vi "Handle Error.vi"(8 "error in (no error)":errorcluster, 11 "cRIO-CO2 in":refnum<class "cRIO-CO2.lvclass">) -> (0 "error out":errorcluster, 2 "stop actor?":bool=TRUE, 3 "cRIO-CO2 out":refnum<class "cRIO-CO2.lvclass">)   [LabVIEW 2015, in "cRIO-Carbondioxide.lvlib" / "cRIO-CO2.lvlib" / "cRIO-CO2.lvclass"]
doc: "(<B>Filename</B>: Actor Framework.lvlib:Actor.lvclass:Handle Error.vi)\n\nDefines how the actor handles an error that occurred while processing a message.\n\nBy default, this method does nothing except stop the actor. This method also treats error code 43 (coming from <B>error in</B>) as a sign that the actor shut down normally. In this situation, the Handle Error method does not return the error on <B>error out</B>, meaning the actor's caller will not receive it. All other error codes will be returned on <B>error out</B>.\n\nA descendant class may override this method to change this behavior."
uses:
  cRIO-CO2.lvclass
  cRIO-CO2.lvclass/cRIO-CO2.ctl
  cRIO-CO2 Messages/Log Error Msg/Log Error Msg.lvclass/Log Error Msg.ctl
  <vilib>/ActorFramework/Message Enqueuer/Message Enqueuer.lvclass/Message Enqueuer.ctl
  <vilib>/ActorFramework/Message Enqueuer/Enqueue.vi
  <vilib>/ActorFramework/Message Priority Queue/Priority Enqueue.vi
  cRIO-CO2 Messages/Log Error Msg/Log Error Msg.lvclass
  <vilib>/ActorFramework/Actor/Actor.lvclass
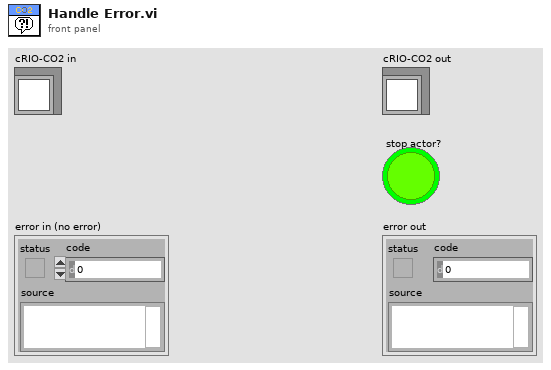
[diagram p1: front panel]
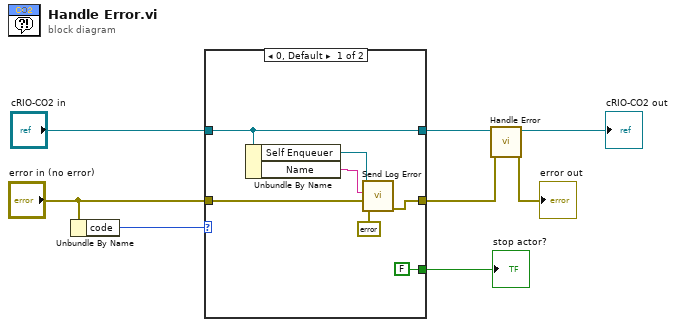
[diagram p0: block diagram]
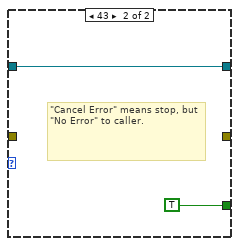
[diagram p2: hidden frame]
diagram:
  n1 = Unbundle By Name("error in (no error)") -> ("code"=w1:i32)
  n2 = case shown="0, Default" w1 {
    tunnel: "cRIO-CO2 in" -> [w11 w17]
    tunnel: [w11 w17] -> w5
    tunnel: [w9 _] -> w4
    tunnel: "error in (no error)" -> [w10 _]
    tunnel: [FALSE ("stop actor?") TRUE ("stop actor?")] -> w2
    frame 0, Default {
      n3 = Unbundle By Name(w11) -> ("Self Enqueuer"=w13:refnum<class "Message Enqueuer.lvclass">, "Name"=w12:string)
      n4 = call "Send Log Error.vi"("error in (no error)"=errorcluster {"status"=FALSE, "code"=0, "source"=""}, "error to log (no error)"=w10, "Source Name"=w12, "Message Enqueuer"=w13) -> ("error out"=w9:errorcluster)  [unwired: 6 in, 1 out]
    }
    frame 43 {
      # "\"Cancel Error\" means stop, but \"No Error\" to caller."
    }
  }
  "stop actor?" <- w2
  n5 = call-parent "Handle Error.vi"("error in (no error)"=w4, "Actor in"=w5) -> ("error out"=→"error out":errorcluster, "Actor out"=→"cRIO-CO2 out":refnum<class "cRIO-CO2.lvclass">)  [unwired: 7 in, 1 out]
